vi "Find Control Refs.vi"(9 "Label.Text Filter":string[](array[string]), 10 "Control Types":string[](array[string]), 11 "Pane Reference In":refnum<vi>) -> (1 "Control Indicies":i32[](array[numeric]), 2 "Control Refs":refnum<vi>[](array[refnum]), 3 "Pane Reference Out (Dup)":refnum<vi>)   [LabVIEW 2019, in "User Interface.lvlib"]
doc: "Takes in a Pane reference and finds all of the controls according to the Class Names input. If any control labels contain the text in Label.Text Filter, they are not included in the output Control Refs array.\n\nThe Control Indicies array elements map directly to the Control Refs array elements. Side note: Control Index values are set by changing the tab order of a front panel."
uses:
  User Interface.lvlib
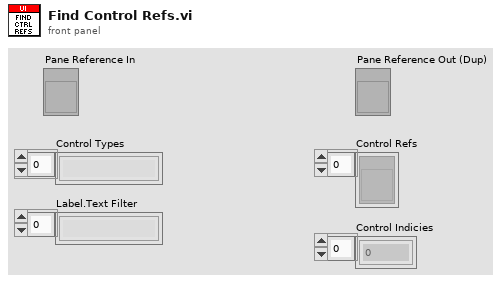
[diagram p1: front panel]
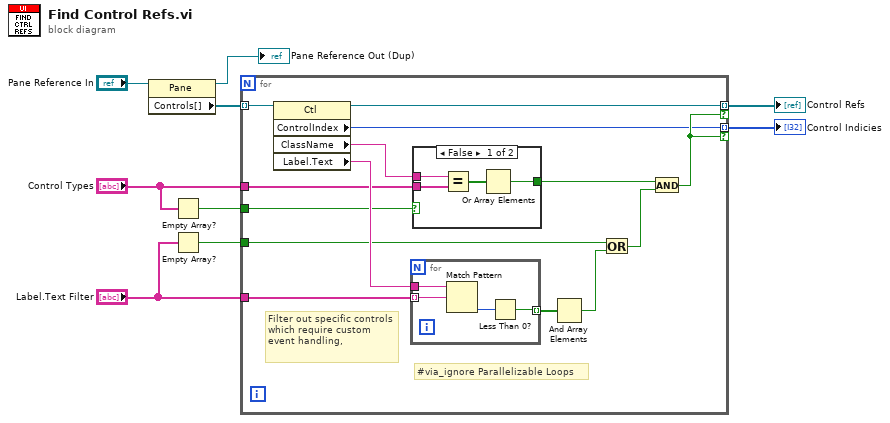
[diagram p0: block diagram]
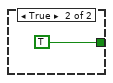
[diagram p2: hidden frame]
diagram:
  n1 = property class="Pane"(reference="Pane Reference In") -> (reference out=→"Pane Reference Out (Dup)":refnum<vi>, "Controls[]"=w9:refnum<vi>[])  [unwired: 1 in, 1 out]
  n2 = Empty Array?(array="Control Types") -> (empty?=w5:bool)
  n3 = Empty Array?(array="Label.Text Filter") -> (empty?=w3:bool)
  n4 = for {
    tunnel: w9 -> [w23] mode=indexing
    tunnel: [w18] -> w7 mode=indexing if=w11
    tunnel: "Label.Text Filter" -> [w17]
    tunnel: "Control Types" -> [w16]
    tunnel: w5 -> [w15]
    tunnel: w3 -> [w14]
    tunnel: [w10] -> w1 mode=indexing if=w11
    # "#via_ignore Parallelizable Loops"
    # "Filter out specific controls which require custom event handling,"
    n5 = property class="Ctl"(reference=w23) -> (reference out=w18:refnum<vi>, "ControlIndex"=w10:i32, "ClassName"=w22:string, "Label.Text"=w19:string)  [unwired: 1 in, 1 out]
    n6 = for {
      tunnel: w19 -> [w32]
      tunnel: w17 -> [w31] mode=indexing
      tunnel: [w29] -> w21 mode=indexing
      n7 = Match Pattern(string=w32, regular expression=w31) -> (offset past match=w30:i32)  [unwired: 1 in, 3 out]
      n8 = Less Than 0?(x=w30) -> (x < 0?=w29:bool)
    }
    n9 = case shown="False" w15 {
      tunnel: w22 -> [w26 _]
      tunnel: [w25 TRUE] -> w20
      tunnel: w16 -> [w24 _]
      frame False {
        n10 = Equal?(x=w26, y=w24) -> (x = y?=w27:bool[])
        n11 = Or Array Elements(Boolean array=w27) -> (logical OR=w25:bool)
      }
      frame True {
      }
    }
    n12 = And Array Elements(Boolean array=w21) -> (logical AND=w13:bool)
    n13 = Or(x=w14, y=w13) -> (x .or. y?=w12:bool)
    n14 = And(x=w20, y=w12) -> (x .and. y?=w11:bool)
  }
  "Control Refs" <- w7
  "Control Indicies" <- w1
